vi "sv_Uniquify SubString.vi"(9 "separator":string="_", 10 "reserved strings":string[](array[string]), 11 "substring":string) -> (1 "uniquifier":string, 2 "unique increment":u64, 3 "unique string":string)   [LabVIEW 2017]
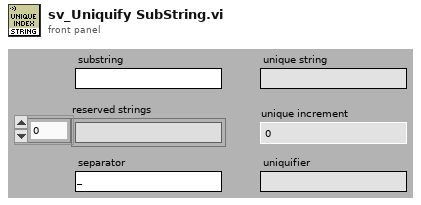
[diagram p1: front panel]
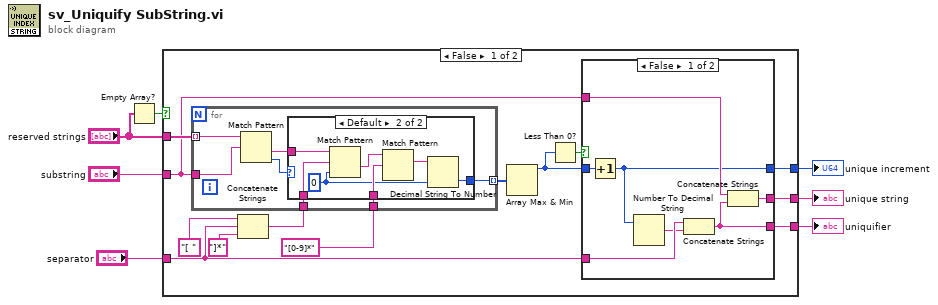
[diagram p0: block diagram]
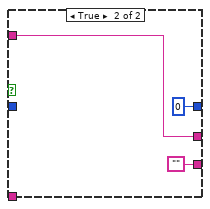
[diagram p2: hidden frame]
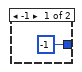
[diagram p3: hidden frame]
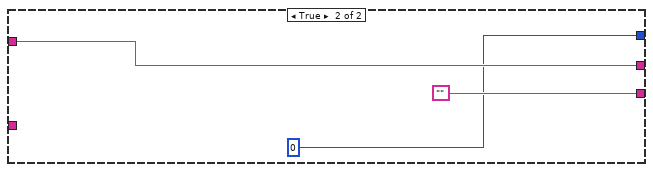
[diagram p4: hidden frame]
diagram:
  n1 = Empty Array?(array="reserved strings") -> (empty?=w5:bool)
  n2 = case shown="False" w5 {
    tunnel: "substring" -> [w15 w48]
    tunnel: "reserved strings" -> [w20 _]
    tunnel: [w18 ""] -> w6
    tunnel: [w16 w48] -> w3
    tunnel: [w17 u64 0 ("unique increment")] -> w2
    tunnel: "separator" -> [w14 _]
    frame False {
      n3 = Concatenate Strings("[ " ("string"), w14, "]*" ("string")) -> (w11:string)
      n4 = for {
        tunnel: w20 -> [w37] mode=indexing
        tunnel: w15 -> [w36]
        tunnel: [w33] -> w19 mode=indexing
        tunnel: w11 -> [w32]
        tunnel: "[0-9]*" ("regular expression") -> [w31]
        n5 = Match Pattern(string=w37, regular expression=w36) -> (after substring=w34:string, offset past match=w35:i32)  [unwired: 1 in, 2 out]
        n6 = case shown="Default" w35 {
          tunnel: w34 -> [_ w45]
          tunnel: [i64 -1 w44] -> w33
          tunnel: w32 -> [_ w43]
          tunnel: w31 -> [_ w41]
          frame -1 {
          }
          frame Default {
            w40 = i64 0 ("offset (0)")
            n7 = Match Pattern(string=w45, regular expression=w43, offset (0)=w40) -> (after substring=w42:string)  [unwired: 3 out]
            n8 = Match Pattern(string=w42, regular expression=w41) -> (match substring=w39:string)  [unwired: 1 in, 3 out]
            n9 = Decimal String To Number(string=w39, default (0L)=w40) -> (number=w44:i64)  [unwired: 1 in, 1 out]
          }
        }
      }
      n10 = Array Max & Min(array=w19) -> (max value=w8:i64)  [unwired: 3 out]
      n11 = Less Than 0?(x=w8) -> (x < 0?=w9:bool)
      n12 = case shown="False" w9 {
        tunnel: [w22 ""] -> w18
        tunnel: [w24 u64 0] -> w17
        tunnel: [w25 w29] -> w16
        tunnel: w15 -> [w26 w29]
        tunnel: w14 -> [w27 _]
        tunnel: w8 -> [w21 _]
        frame False {
          n13 = Increment(x=w21) -> (x+1=w24:i64)
          n14 = Number To Decimal String(number=w24) -> (decimal integer string=w23:string)  [unwired: 1 in]
          n15 = Concatenate Strings(w27, w23) -> (w22:string)
          n16 = Concatenate Strings(w26, w22) -> (w25:string)
        }
        frame True {
        }
      }
    }
    frame True {
    }
  }
  "unique string" <- w3
  "uniquifier" <- w6
  "unique increment" <- w2
